vi "Shut Down Flash Cameras.vi"(8 "error in (no error)":errorcluster, 11 "Virtual Camera in":refnum<class "Virtual Camera.lvclass">) -> (0 "error out":errorcluster, 3 "Virtual Camera out":refnum<class "Virtual Camera.lvclass">)   [LabVIEW 2017, in "Virtual Camera.lvlib" / "Virtual Camera.lvclass"]
uses:
  Virtual Camera.lvclass
  Virtual Camera.lvclass/Virtual Camera.ctl
  <vilib>/ActorFramework/Message Enqueuer/Message Enqueuer.lvclass/Message Enqueuer.ctl
  <vilib>/ActorFramework/Message Enqueuer/Enqueue.vi
  <vilib>/ActorFramework/Stop Msg/Stop Msg.lvclass
  C:/Program Files/National Instruments/LabVIEW 2017/vi.lib/ActorFramework/Message/Message.lvclass
  Resources/GLOBAL/GLOBAL Time-critical.vi
  <vilib>/ActorFramework/Message Priority Queue/Priority Enqueue.vi
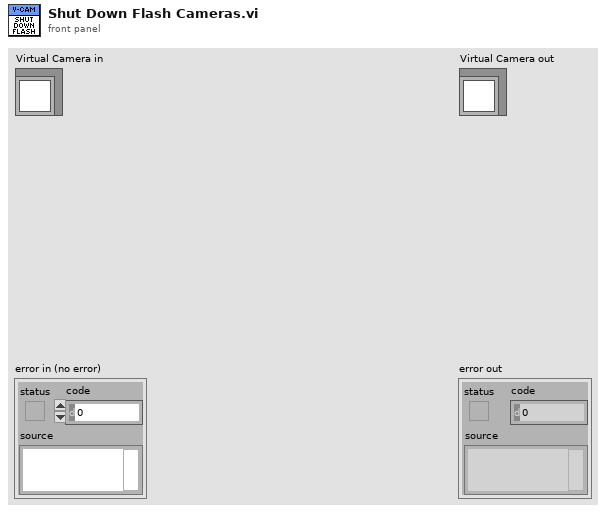
[diagram p1: front panel]
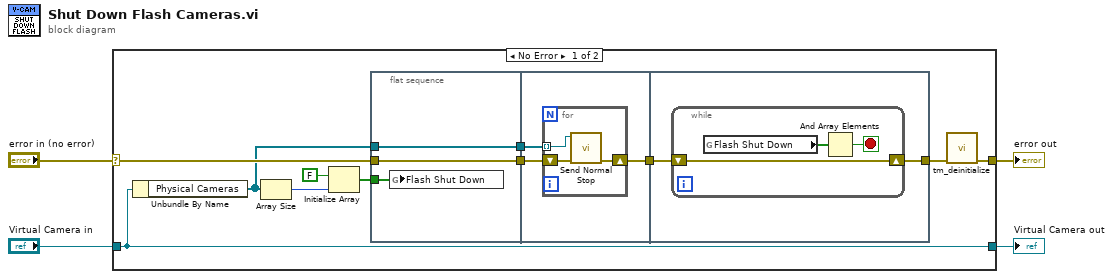
[diagram p0: block diagram]
diagram:
  n1 = case shown="No Error" "error in (no error)" {
    selector: "error in (no error)" -> [w14 w31]
    tunnel: [w13 w31] -> w3
    tunnel: [w15 w30] -> w1
    tunnel: "Virtual Camera in" -> [w15 w30]
    frame No Error {
      n2 = Unbundle By Name(w15) -> ("Physical Cameras"=w10:refnum<class "Message Enqueuer.lvclass">[])
      n3 = Array Size(array=w10) -> (size(s)=w9:i32)
      n4 = Initialize Array(FALSE, w9) -> (w8:bool[])
      n5 = flat-sequence {
        tunnel: w10 -> [w17]
        tunnel: w14 -> [w18]
        tunnel: [w18] -> w12
        tunnel: [w17] -> w11
        tunnel: w8 -> [w16]
        tunnel: w12 -> [w21]
        tunnel: w11 -> [w20]
        tunnel: [w19] -> w6
        tunnel: w6 -> [w26]
        tunnel: [w25] -> w5
        frame #0 {
          n6 = global write "GLOBAL Time-critical.vi" "Flash Shut Down"(w16) -> ()
        }
        frame #1 {
          n7 = for {
            tunnel: w20 -> [w22] mode=indexing
            shift-right: [w23] -> w19
            shift-left: w21 -> [w24]
            n8 = call <vilib>:"Send Normal Stop.vi"("error in (no error)"=w24, "Message Enqueuer"=w22) -> ("error out"=w23:errorcluster)  [unwired: 9 in]
          }
        }
        frame #2 {
          n9 = while {
            shift-right: [w27] -> w25
            shift-left: w26 -> [w27]
            stop <- w28 stop-if-true
            n10 = global read "GLOBAL Time-critical.vi" "Flash Shut Down"() -> (w29:bool[])
            n11 = And Array Elements(Boolean array=w29) -> (logical AND=w28:bool)
          }
        }
      }
      n12 = call <userlib>:"tm_deinitialize.vi"("error in (no error)"=w5) -> ("error out"=w13:errorcluster)  [unwired: 10 in]
    }
    frame Error {
    }
  }
  "error out" <- w3
  "Virtual Camera out" <- w1
